vi "Read Default Value.vi"(8 "error in":errorcluster, 11 "analog channel in":refnum<class "Analog Channel.lvclass">) -> (0 "error out":errorcluster, 2 "default value":dbl, 3 "analog channel out":refnum<class "Analog Channel.lvclass">)   [LabVIEW 2017, in "Analog Channel.lvclass"]
uses:
  Analog Channel.lvclass
  Analog Channel.lvclass/Analog Channel.ctl
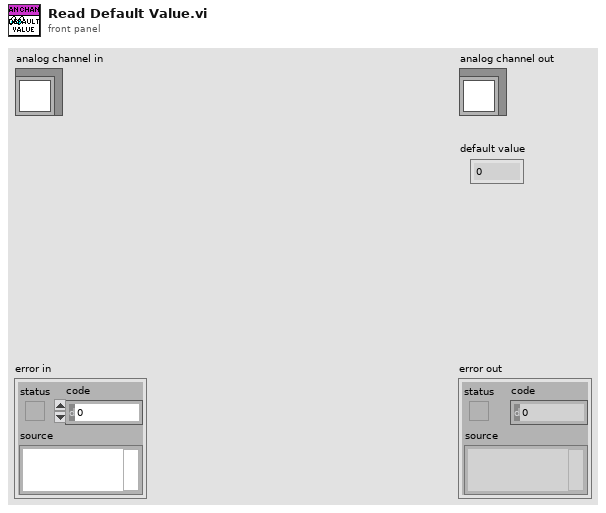
[diagram p1: front panel]
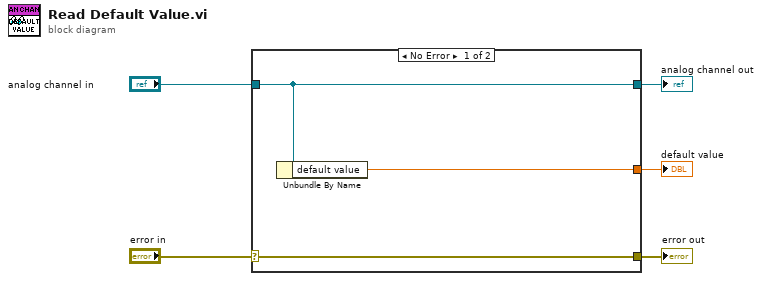
[diagram p0: block diagram]
diagram:
  n1 = case shown="No Error" "error in" {
    selector: "error in" -> [w8 w9]
    tunnel: [w8 w9] -> w4
    tunnel: [w7 w10] -> w2
    tunnel: "analog channel in" -> [w7 w10]
    tunnel: [w6 _] -> w1
    frame No Error {
      n2 = Unbundle By Name(w7) -> ("default value"=w6:dbl)
    }
    frame Error {
    }
  }
  "error out" <- w4
  "analog channel out" <- w2
  "default value" <- w1
